vi "Add Rx UDP VLs and UDPs.vi"(8 "error in":errorcluster, 10 "Rx UDP configuration":T7(array[cluster]) {"sapPorts"."Parameters"."Parameter"."encoding" items=["BNR", "BCD", "Discrete", "Signed_32", "Signed_64", "Float_32", "Float_64", "Opaque"]; "commPorts"."Parameters"."Parameter"."encoding" items=["BNR", "BCD", "Discrete", "Signed_32", "Signed_64", "Float_32", "Float_64", "Opaque"]; "Tx_UDP"."FilterMode" items=["FDX_RX_VL_FLT_DIS", "FDX_RX_VL_FLT_ENA ", "FDX_RX_VL_FLT_ENA_INV"]; "Tx_UDP"."VLBufSize" format="%.0x"; "Tx_UDP"."VerificationMode" items=["FDX_RX_VL_CHECK_ENA_DEFAULT"=65535, "FDX_RX_VL_CHECK_REDMAM"=16, "DX_RX_VL_CHECK_TRAFIC"=8, "FDX_RX_VL_CHECK_FRAMESIZE"=4, "FDX_RX_VL_CHECK_SNINTEG"=2, "FDX_RX_VL_CHECK_INVPAC"=1, "FDX_RX_VL_CHECK_DISA"=0]}, 11 "Rx UDP ref":T8 format="%.0x") -> (0 "error out":errorcluster, 3 "Rx UDP ref out":T8 format="%.0x")   [LabVIEW 2020, in "AIM ARINC 664 Scripting.lvlib"]
doc: "Add Rx UPD VLs, UDP ports and parameters based on the Tx UDP configuration."
uses:
  AIM ARINC 664 Scripting.lvlib
  <vilib>/NI VeriStand/Custom Device API/Custom Device Item Ref.ctl
  Import/_typedefs/rx_udp_setup.ctl
  Import/_typedefs/port_rx_udp_comm.ctl
  Import/_typedefs/frame_parameter.ctl
  Import/_typedefs/frame_parameter_definition.ctl
  Shared/Encoding (Arinc664).ctl
  Import/_typedefs/port_rx_udp_sap.ctl
  <instrlib>/AIM GmbH/_AIM 664/_controls/comm_verification_rx.ctl
  <instrlib>/AIM GmbH/_AIM 664/_controls/comm_udp_rx.ctl
  <vilib>/NI VeriStand/Custom Device API/Custom Device Channel Type.ctl
  Constants.vi
  <vilib>/NI VeriStand/Custom Device API/Custom Device API.lvlib
  <instrlib>/AIM GmbH/_AIM 664/AIM664LV.lvlib
  Import/AIM ARINC 664 Import.lvlib
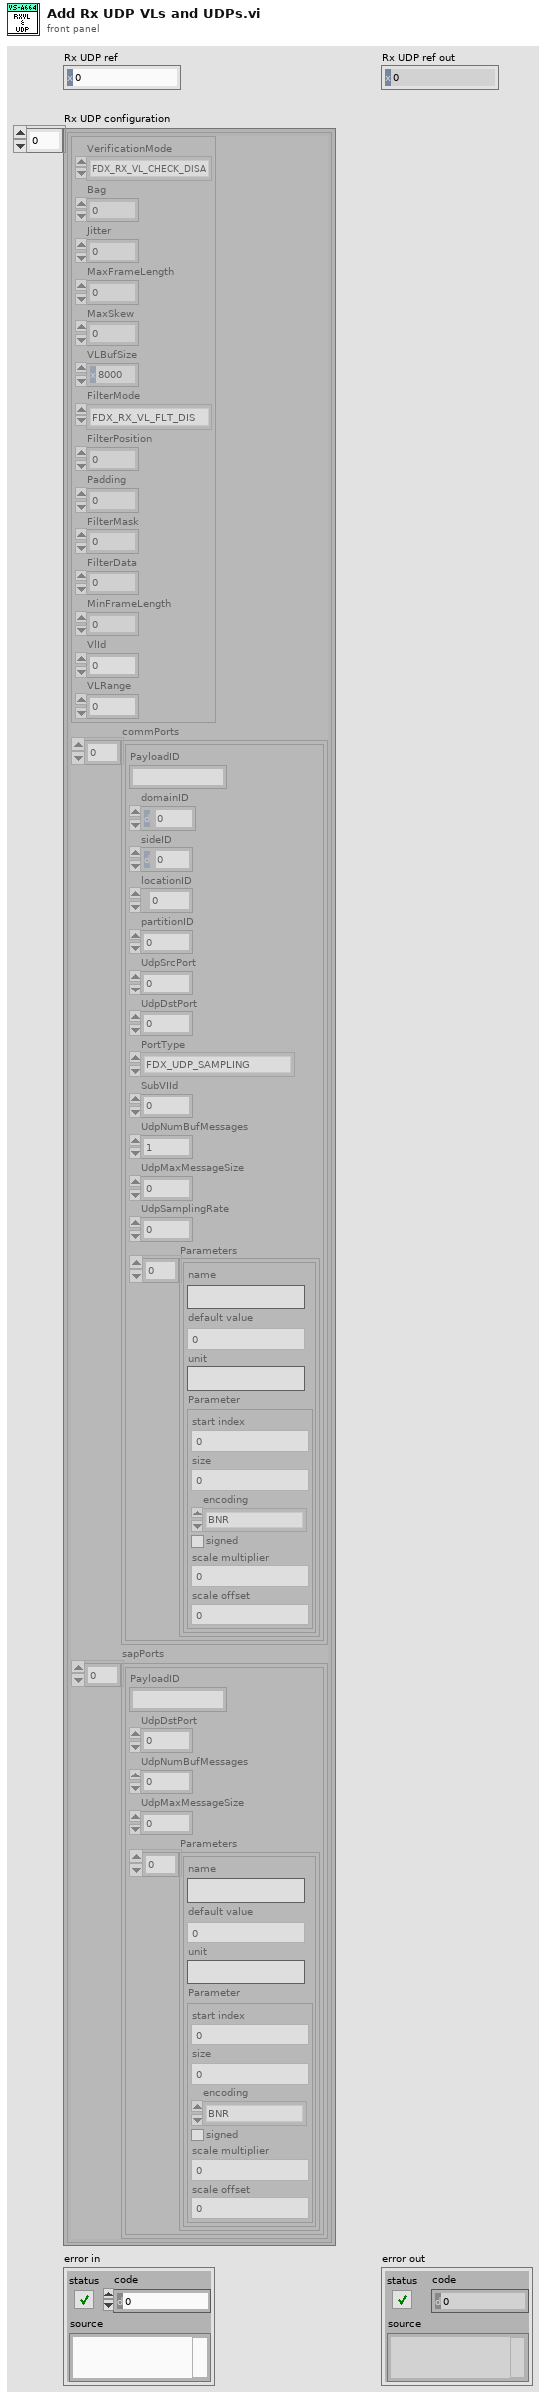
[diagram p1: front panel]
types:
  T1 = typedef "AIM ARINC 664 Import.lvlib/rx_udp_setup.ctl" = cluster{"VerificationMode":u32, "Bag":u32, "Jitter":u32, "MaxFrameLength":u32, "MaxSkew":u32, "VLBufSize":u32, "FilterMode":u32, "FilterPosition":u32, "Padding":u32, "FilterMask":u32, "FilterData":u32, "MinFrameLength":u32, "VlId":u16, "VLRange":u32}
  T2 = typedef "AIM ARINC 664 Import.lvlib/port_rx_udp_comm.ctl" = cluster{"PayloadID":string, "domainID":u8, "sideID":u8, "locationID":u8, "partitionID":u8, "UdpSrcPort":u16, "UdpDstPort":u16, "PortType":enum16{"FDX_UDP_SAMPLING", "FDX_UDP_QUEUING"}, "SubVIId":u32, "UdpNumBufMessages":u32, "UdpMaxMessageSize":u32, "UdpSamplingRate":u32, "Parameters":T3[]}
  T3 = typedef "AIM ARINC 664 Import.lvlib/frame_parameter.ctl" = cluster{"name":string, "default value":dbl, "unit":string, "Parameter":T4}
  T4 = typedef "AIM ARINC 664 Import.lvlib/frame_parameter_definition.ctl" = cluster{"start index":i32, "size":i32, "encoding":T5, "signed":bool, "scale multiplier":dbl, "scale offset":dbl}
  T5 = typedef "Encoding (Arinc664).ctl" = u16
  T6 = typedef "AIM ARINC 664 Import.lvlib/port_rx_udp_sap.ctl" = cluster{"PayloadID":string, "UdpDstPort":u16, "UdpNumBufMessages":u32, "UdpMaxMessageSize":u32, "Parameters":T3[]}
  T7 = cluster{"Tx_UDP":T1, "commPorts":T2[], "sapPorts":T6[]}[]
  T8 = typedef "Custom Device API.lvlib/Custom Device Item Ref.ctl" = u64
  T9 = typedef "AIM664LV.lvlib/comm_verification_rx.ctl" = cluster{"VlId":u16, "VLRange":u32, "VerificationMode":u32, "Bag":u32, "Jitter":u32, "MaxFrameLength":u32, "MaxSkew":u32, "VLBufSize":u32, "FilterMode":u32, "FilterPosition":u32, "Padding":u32, "FilterMask":u32, "FilterData":u32, "MinFrameLength":u32}
  T10 = typedef "AIM664LV.lvlib/comm_udp_rx.ctl" = cluster{"PortType":enum16{"FDX_UDP_SAMPLING", "FDX_UDP_QUEUING"}, "SubVIId":u32, "domainID":u8, "sideID":u8, "locationID":u8, "partitionID":u8, "UdpSrcPort":u16, "UdpDstPort":u16, "UdpNumBufMessages":u32, "UdpMaxMessageSize":u32, "UdpSamplingRate":u32}
  T11 = typedef "Custom Device API.lvlib/Custom Device Channel Type.ctl" = enum16{"Input", "Output"}
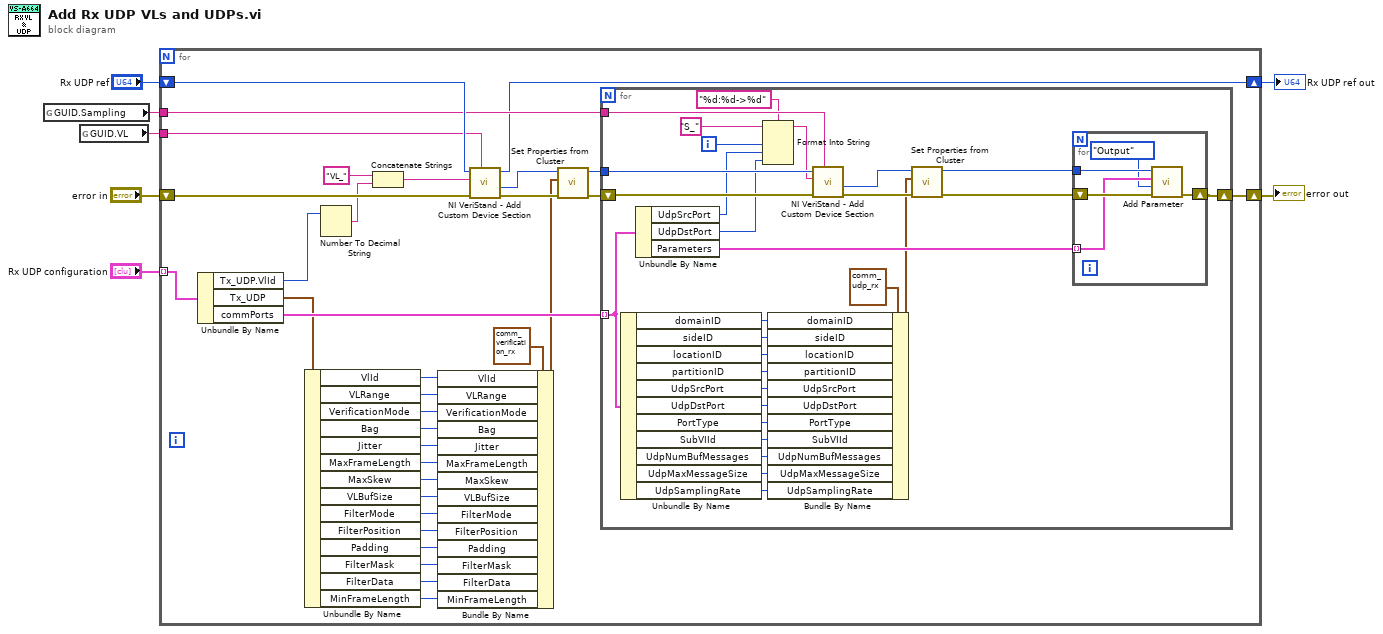
[diagram p0: block diagram]
diagram:
  n1 = global read "Constants.vi" "GUID.Sampling"() -> (w2:string)
  n2 = global read "Constants.vi" "GUID.VL"() -> (w3:string)
  n3 = for {
    tunnel: "Rx UDP configuration" -> [w27] mode=indexing
    shift-right: [w25] -> w1
    shift-left: "Rx UDP ref" -> [w40]
    shift-right: [w38] -> w4
    shift-left: "error in" -> [w39]
    tunnel: w3 -> [w33]
    tunnel: w2 -> [w32]
    n4 = Unbundle By Name(w27) -> ("Tx_UDP.VlId"=w31:u16, "Tx_UDP"=w23:T1, "commPorts"=w34:T2[])
    n5 = Unbundle By Name(w23) -> ("VlId"=w21:u16, "VLRange"=w20:u32, "VerificationMode"=w19:u32, "Bag"=w18:u32, "Jitter"=w17:u32, "MaxFrameLength"=w16:u32, "MaxSkew"=w15:u32, "VLBufSize"=w14:u32, "FilterMode"=w13:u32, "FilterPosition"=w12:u32, "Padding"=w11:u32, "FilterMask"=w10:u32, "FilterData"=w9:u32, "MinFrameLength"=w8:u32)
    n6 = Number To Decimal String(number=w31) -> (decimal integer string=w36:string)  [unwired: 1 in]
    n7 = Concatenate Strings("VL_" ("string"), w36) -> (w35:string)
    n8 = Bundle By Name(cluster=T9 {"VlId"=0, "VLRange"=0, "VerificationMode"=0, "Bag"=0, "Jitter"=0, "MaxFrameLength"=0, "MaxSkew"=0, "VLBufSize"=32768, "FilterMode"=0, "FilterPosition"=0, "Padding"=0, "FilterMask"=0, "FilterData"=0, "MinFrameLength"=0} ("VL Config"), "VlId"=w21, "VLRange"=w20, "VerificationMode"=w19, "Bag"=w18, "Jitter"=w17, "MaxFrameLength"=w16, "MaxSkew"=w15, "VLBufSize"=w14, "FilterMode"=w13, "FilterPosition"=w12, "Padding"=w11, "FilterMask"=w10, "FilterData"=w9, "MinFrameLength"=w8) -> (w22:T9)
    n9 = call <vilib>:"NI VeriStand - Add Custom Device Section.vi"("GUID (Default Section)"=w33, "error in (no error)"=w39, "Section Name"=w35, "Parent Ref in"=w40) -> ("error out"=w29:errorcluster, "Section Ptr"=w30:T8, "Parent Ref out"=w25:T8)  [unwired: 4 in, 1 out]
    n10 = call "Set Properties from Cluster.vi"("error in"=w29, "Variant Cluster"=w22, "item ref in"=w30) -> ("error out"=w28:errorcluster, "item ref out"=w26:T8)  [unwired: 7 in]
    n11 = for {
      shift-right: [w65] -> w38
      shift-left: w28 -> [w68]
      tunnel: w34 -> [w56] mode=indexing
      tunnel: w32 -> [w67]
      tunnel: w26 -> [w69]
      i -> [w63]
      n12 = Unbundle By Name(w56) -> ("domainID"=w54:u8, "sideID"=w53:u8, "locationID"=w52:u8, "partitionID"=w51:u8, "UdpSrcPort"=w50:u16, "UdpDstPort"=w49:u16, "PortType"=w48:enum16{"FDX_UDP_SAMPLING", "FDX_UDP_QUEUING"}, "SubVIId"=w47:u32, "UdpNumBufMessages"=w46:u32, "UdpMaxMessageSize"=w45:u32, "UdpSamplingRate"=w44:u32)
      n13 = Unbundle By Name(w56) -> ("UdpSrcPort"=w61:u16, "UdpDstPort"=w60:u16, "Parameters"=w66:T3[])
      n14 = Format Into String(format string="%d:%d->%d", initial string="S_" ("string"), w63, w61, w60) -> (resulting string=w59:string)  [unwired: 1 in, 1 out]
      n15 = Bundle By Name(cluster=T10 {"PortType"=enum."FDX_UDP_SAMPLING", "SubVIId"=0, "domainID"=1, "sideID"=1, "locationID"=1, "partitionID"=1, "UdpSrcPort"=0, "UdpDstPort"=0, "UdpNumBufMessages"=0, "UdpMaxMessageSize"=0, "UdpSamplingRate"=0} ("CommPort Config"), "domainID"=w54, "sideID"=w53, "locationID"=w52, "partitionID"=w51, "UdpSrcPort"=w50, "UdpDstPort"=w49, "PortType"=w48, "SubVIId"=w47, "UdpNumBufMessages"=w46, "UdpMaxMessageSize"=w45, "UdpSamplingRate"=w44) -> (w55:T10)
      n16 = call <vilib>:"NI VeriStand - Add Custom Device Section.vi"("GUID (Default Section)"=w67, "error in (no error)"=w68, "Section Name"=w59, "Parent Ref in"=w69) -> ("error out"=w57:errorcluster, "Section Ptr"=w58:T8)  [unwired: 4 in, 2 out]
      n17 = call "Set Properties from Cluster.vi"("error in"=w57, "Variant Cluster"=w55, "item ref in"=w58) -> ("error out"=w41:errorcluster, "item ref out"=w42:T8)  [unwired: 7 in]
      n18 = for {
        tunnel: w42 -> [w74]
        tunnel: w66 -> [w72] mode=indexing
        shift-right: [w71] -> w65
        shift-left: w41 -> [w73]
        n19 = call "Add Parameter.vi"("error in (no error)"=w73, "Type (Output)"=Custom_Device_Channel_Type."Output", "parameter"=w72, "section ref in"=w74) -> ("error out"=w71:errorcluster)  [unwired: 6 in, 1 out]
      }
    }
  }
  "Rx UDP ref out" <- w1
  "error out" <- w4
